vi "CCEditDicomTags.vi"(10 "Table":string[][](table)=[[""]], 11 "RowNames":string[](array[string])) -> (2 "Cancel?":bool, 3 "TableOut":string[][](table))   [LabVIEW 2013, in "ClearCanvasLibrary.lvlib"]
uses:
  ClearCanvasLibrary.lvlib
  main.lvlib
  Controls/Enum Save Action Events.ctl
  Controls/Enum Variables.ctl
  Controls/Enum DICOM.ctl
panel:
  in  "Down Button":bool
  in  "Up Button":bool
  in  "DicomEditCancelBtn":bool
  in  "DicomEditSaveBtn":bool
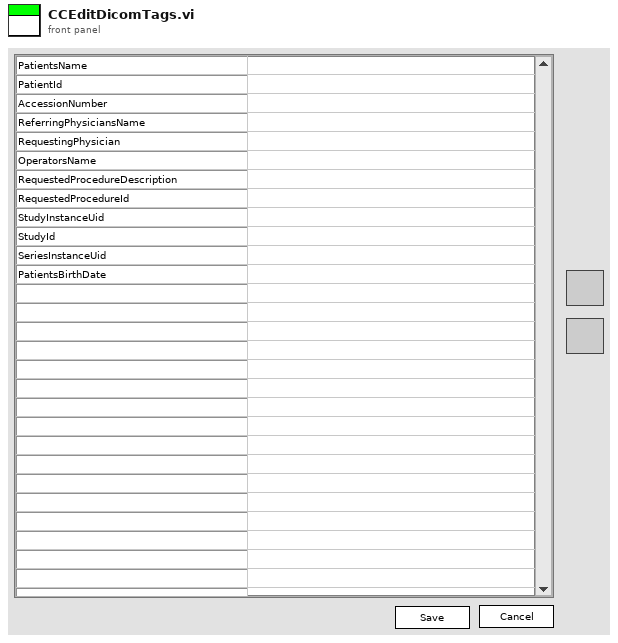
[diagram p1: front panel]
types:
  T1 = typedef "LVRowAndColumnTypeDef.ctl" = cluster{"Row":i32, "Column":i32}
  T2 = typedef "main.lvlib/Enum DICOM.ctl" = enum16{"Set DICOM itemTags", "Set Dicom Encoding", "Set DICOM Attributes"}
  T3 = typedef "main.lvlib/Enum Variables.ctl" = enum16{"SetAcqFilter", "GetAcqFilter", "Set Filter", "Get Filter", "Set Height", "Get Height", "Set Blue Pressure", "Get Blue Pressure", "Set Red Pressure", "Get Red Pressure", "Init", "Reset Pressure", "Set Red Cursors", "Get Red Cursors", "Set Blue Cursors", "Get Blue Cursors", "Set Language", "Get Language", "Set Active Graphs", "Get ActiveGraphs", "Set Method", "Get Method", "Set Encryption", "Get Encryption", "Set ExcelVersion", "Get ExcelVersion", "Set DICOM Avail", "Get DICOM Avail", "Set DICOM Encode", "Get DICOM Encode", "Set JournalExport", "Get JournalExport", "Set Sequence", "Get Sequence", "Set DAQ Connected", "Get DAQ Connected", "Set Current Graph", "Get Current Graph", "Set General Settings", "Get Hyphenation", "Set Arm Calc Method", "Get Arm Calc Method", "Set Dicom Tags", "Get Dicom Tags", "Set BT Serial", "Get BT Serial", "Set BT Accepted Serials", "Get BT Accepted Serials", "Get BT License", "Set BT License"}
  T4 = typedef "main.lvlib/Enum Save Action Events.ctl" = enum16{"LoadReportPath", "SaveReportPath", "Load Graph Path", "Save Graph Path", "LoadDataPath", "SaveDataPath", "Load Template Path", "Save Template Path", "Load PressureFactor", "Save PressureFactor", "Init", "Load Listbox", "Save Listbox", "LoadHospInfo", "SaveHospInfo", "Load DICOM Activation", "Save DICOM Activation", "LoadDICOMInfoWL", "SaveDICOMInfoWL", "LoadDICOMInfoPACS", "SaveDICOMInfoPACS", "Load ArmCalcMethod", "Save ArmCalcMethod", "LoadItemTags", "SaveItemTags", "LoadDICOMEncoding", "SaveDICOMEncoding", "LoadJournalType", "SaveJournalType", "LoadAcqFilterType", "SaveAcqFilterType", "Load Sequence", "Save Sequence", "Load Acquisition Mode", "Save Acquisition Mode", "Load General Settings", "Save General Settings", "Load Language", "Save Language", "Load Dicom Tags", "Save Dicom Tags", "Load BT Serial", "Save BT Serial", "Load BT License", "Save BT License"}
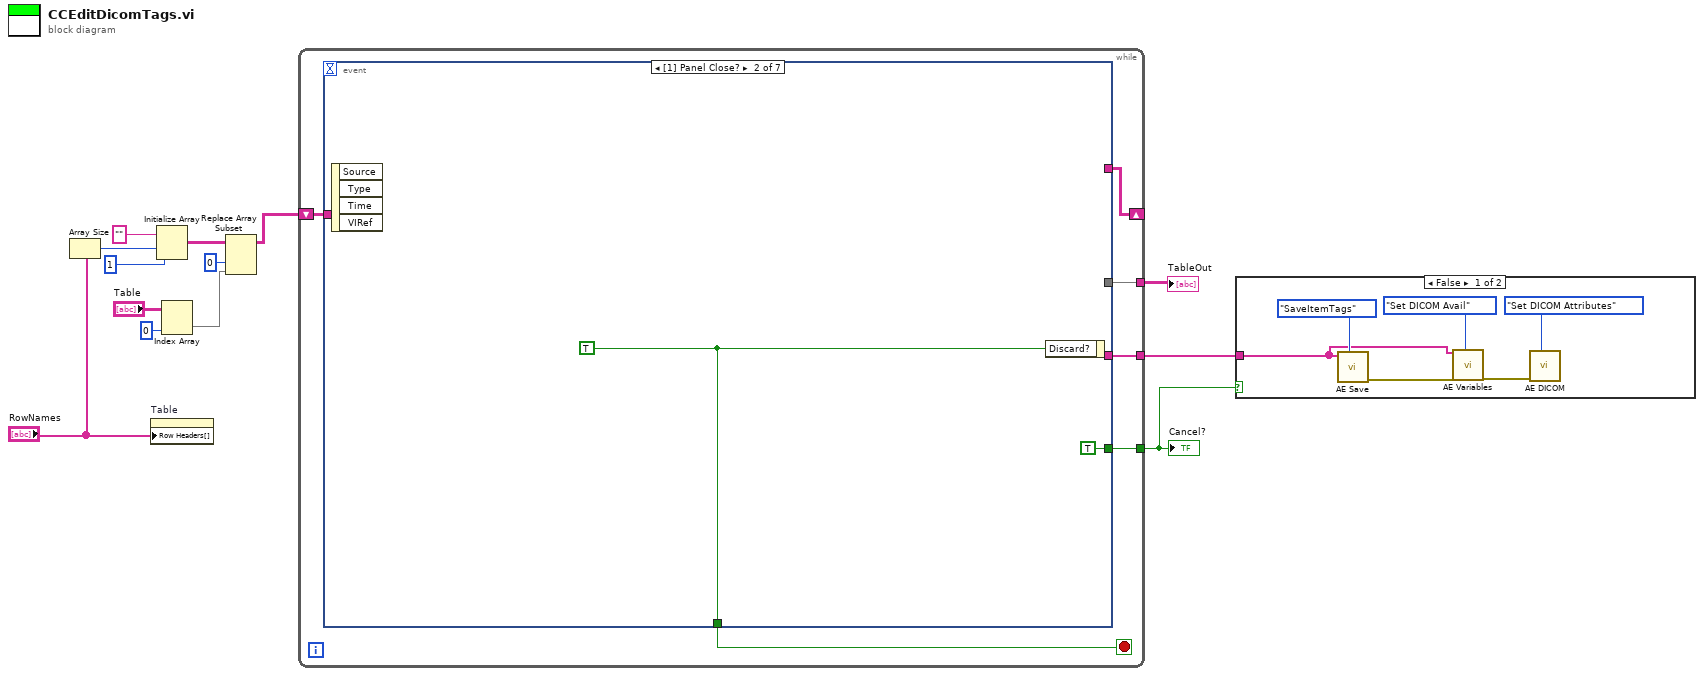
[diagram p0: block diagram]
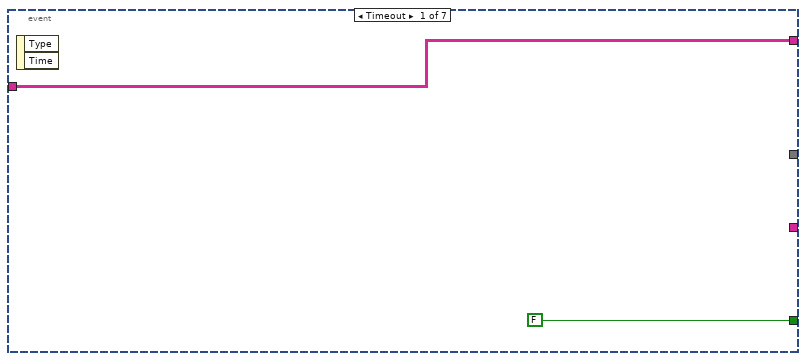
[diagram p3: hidden frame]
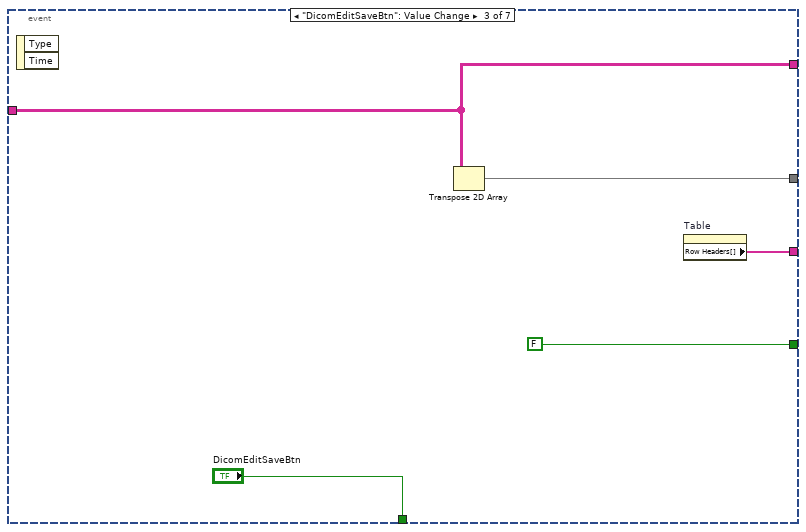
[diagram p4: hidden frame]
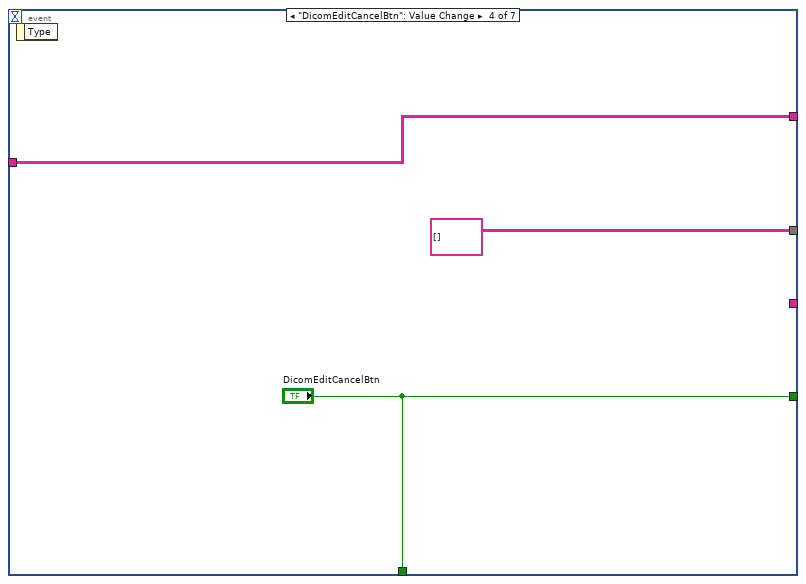
[diagram p5: hidden frame]
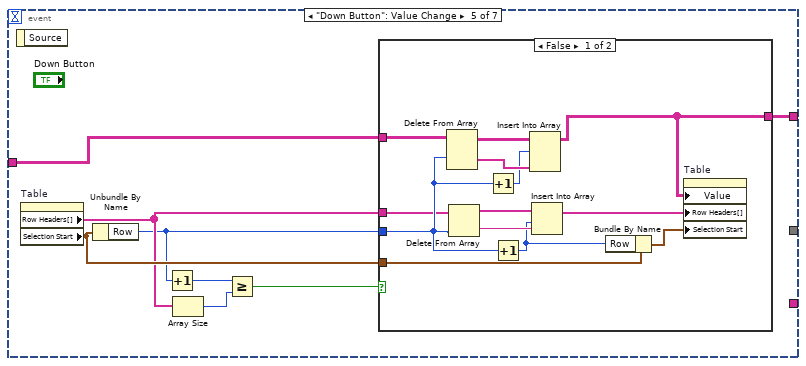
[diagram p6: hidden frame]
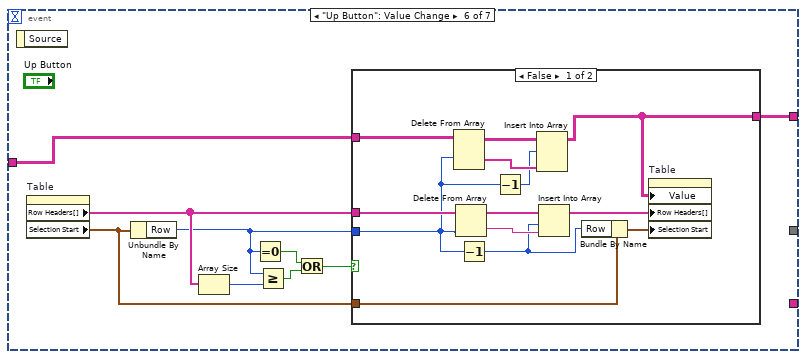
[diagram p8: hidden frame]
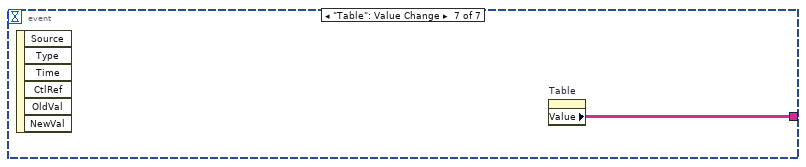
[diagram p10: hidden frame]
diagram:
  n1 = Array Size(array="RowNames") -> (size(s)=w10:i32)
  n2 = property on="Table" class="Tbl (strict)"("Row Headers[]"="RowNames") -> ()  [unwired: 2 in, 2 out]
  n3 = Initialize Array("", w10, 1 ("dimension size")) -> (w9:string[][])
  n4 = Index Array(array="Table", index (col)=0 ("disabled index (col)")) -> (element=w7:string[])  [unwired: 1 in]
  n5 = Replace Array Subset(array=w9, new element=w7, index (col)=0 ("disabled index (col)")) -> (w8:string[][])  [unwired: 1 in]
  n6 = while {
    tunnel: [w18] -> w13
    tunnel: [w17] -> w1
    shift-right: [w15] -> _
    shift-left: w8 -> [w16]
    tunnel: [w14] -> w2
    stop <- w19 stop-if-true
    n7 = event shown="[1] Panel Close?" {
      selector: _ -> [_ _ _ _ _ _ _]
      dyn-events: _ -> [_ _ _ _ _ _ _]
      timeout: _ -> [_ _ _ _ _ _ _]
      tunnel: [_ w23 "DicomEditSaveBtn" "DicomEditCancelBtn" _ _ _] -> w19
      tunnel: [_ _ w27 string[][] [] ("Table") _ _ _] -> w18
      tunnel: [FALSE ("DicomEditCancelBtn") TRUE ("DicomEditCancelBtn") FALSE ("DicomEditCancelBtn") "DicomEditCancelBtn" _ _ _] -> w17
      tunnel: w16 -> [w20 _ w25 w29 w33 w61 _]
      tunnel: [w20 _ w25 w29 w32 w60 w77] -> w15
      tunnel: [_ _ w24 _ _ _ _] -> w14
      event Timeout {
        n8 = event-data() -> ()  [unwired: 1 in, 2 out]
      }
      event Panel Close? {
        w23 = TRUE ("Discard?")
        n9 = event-data() -> ()  [unwired: 1 in, 4 out]
        n10 = event-data("Discard?"=w23) -> ()  [unwired: 1 in, 1 out]
      }
      event "DicomEditSaveBtn": Value Change {
        n11 = event-data() -> ()  [unwired: 1 in, 2 out]
        n12 = Transpose 2D Array(2D array=w25) -> (transposed array=w27:string[][])
        n13 = property on="Table" class="Tbl (strict)"() -> ("Row Headers[]"=w24:string[])  [unwired: 2 in, 2 out]
      }
      event "DicomEditCancelBtn": Value Change {
        n14 = event-data() -> ()  [unwired: 1 in, 1 out]
      }
      event "Down Button": Value Change {
        n15 = event-data() -> ()  [unwired: 1 in, 1 out]
        n16 = property on="Table" class="Tbl (strict)"() -> ("Row Headers[]"=w38:string[], "Selection Start"=w39:T1)  [unwired: 2 in, 2 out]
        n17 = Unbundle By Name(w39) -> ("Row"=w35:i32)
        n18 = Increment(x=w35) -> (x+1=w34:i32)
        n19 = Array Size(array=w38) -> (size(s)=w37:i32)
        n20 = Greater Or Equal?(x=w34, y=w37) -> (x >= y?=w36:bool)
        n21 = case shown="False" w36 {
          tunnel: w33 -> [w52 w53]
          tunnel: w35 -> [w46 _]
          tunnel: w39 -> [w44 _]
          tunnel: w38 -> [w42 _]
          tunnel: [w40 w53] -> w32
          frame False {
            n22 = Delete From Array(array=w52, index (row)=w46) -> (deleted portion=w51:string[], array with subset deleted=w50:string[][])  [unwired: 2 in]
            n23 = Delete From Array(array=w42, index=w46) -> (deleted portion=w48:string, array with subset deleted=w49:string[])  [unwired: 1 in]
            n24 = Increment(x=w46) -> (x+1=w43:i32)
            n25 = Increment(x=w46) -> (x+1=w41:i32)
            n26 = Insert Into Array(array=w50, index (row)=w43, new element=w51) -> (w40:string[][])  [unwired: 1 in]
            n27 = Insert Into Array(array=w49, index=w41, new element=w48) -> (w47:string[])
            n28 = Bundle By Name(cluster=w44, "Row"=w41) -> (w45:T1)
            n29 = property on="Table" class="Tbl (strict)"("Value"=w40, "Row Headers[]"=w47, "Selection Start"=w45) -> ()  [unwired: 2 in, 2 out]
          }
          frame True {
          }
        }
      }
      event "Up Button": Value Change {
        n30 = event-data() -> ()  [unwired: 1 in, 1 out]
        n31 = property on="Table" class="Tbl (strict)"() -> ("Row Headers[]"=w58:string[], "Selection Start"=w62:T1)  [unwired: 2 in, 2 out]
        n32 = Unbundle By Name(w62) -> ("Row"=w57:i32)
        n33 = Array Size(array=w58) -> (size(s)=w59:i32)
        n34 = Equal To 0?(x=w57) -> (x = 0?=w56:bool)
        n35 = Greater Or Equal?(x=w57, y=w59) -> (x >= y?=w55:bool)
        n36 = Or(x=w56, y=w55) -> (x .or. y?=w54:bool)
        n37 = case shown="False" w54 {
          tunnel: w58 -> [w73 _]
          tunnel: w57 -> [w69 _]
          tunnel: w62 -> [w67 _]
          tunnel: w61 -> [w65 w76]
          tunnel: [w63 w76] -> w60
          frame False {
            n38 = Delete From Array(array=w65, index (row)=w69) -> (deleted portion=w75:string[], array with subset deleted=w74:string[][])  [unwired: 2 in]
            n39 = Delete From Array(array=w73, index=w69) -> (deleted portion=w71:string, array with subset deleted=w72:string[])  [unwired: 1 in]
            n40 = Decrement(x=w69) -> (x-1=w64:i32)
            n41 = Decrement(x=w69) -> (x-1=w66:i32)
            n42 = Insert Into Array(array=w74, index (row)=w66, new element=w75) -> (w63:string[][])  [unwired: 1 in]
            n43 = Insert Into Array(array=w72, index=w64, new element=w71) -> (w70:string[])
            n44 = Bundle By Name(cluster=w67, "Row"=w64) -> (w68:T1)
            n45 = property on="Table" class="Tbl (strict)"("Value"=w63, "Row Headers[]"=w70, "Selection Start"=w68) -> ()  [unwired: 2 in, 2 out]
          }
          frame True {
          }
        }
      }
      event "Table": Value Change {
        n46 = event-data() -> ()  [unwired: 1 in, 6 out]
        n47 = property on="Table" class="Tbl (strict)"() -> ("Value"=w77:string[][])  [unwired: 2 in, 2 out]
      }
    }
  }
  "TableOut" <- w13
  "Cancel?" <- w1
  n48 = case shown="False" w1 {
    tunnel: w2 -> [w81 _]
    frame False {
      n49 = call "AE Save.vi"("Variant In"=w81, "Action"=Enum_Save_Action_Events."SaveItemTags") -> ("error out"=w80:errorcluster)  [unwired: 7 in, 1 out]
      n50 = call "AE Variables.vi"("VariantIn"=w81, "error in (no error)"=w80, "Action"=Enum_Variables."Set DICOM Avail") -> ("error out"=w79:errorcluster)  [unwired: 9 in, 7 out]
      n51 = call "AE DICOM.vi"("Action"=Enum_DICOM."Set DICOM Attributes", "Error In"=w79) -> ()  [unwired: 9 in, 1 out]
    }
    frame True {
    }
  }
